vi "Seriennummer zerlegen in Werte.vi"(8 "error in (no error)":errorcluster caption="Fehler (Eingang, kein Fehler)", 10 "Seriennummer":string, 11 "Steuerung PNS Eingang":refnum<class "Steuerung PNS.lvclass">) -> (0 "error out":errorcluster caption="Fehler (Ausgang)", 2 "Werte Array":u16[](array[numeric]), 3 "Steuerung PNS Ausgang":refnum<class "Steuerung PNS.lvclass">)   [LabVIEW 2020, in "Steuerung PNS.lvclass"]
uses:
  Steuerung PNS.lvclass
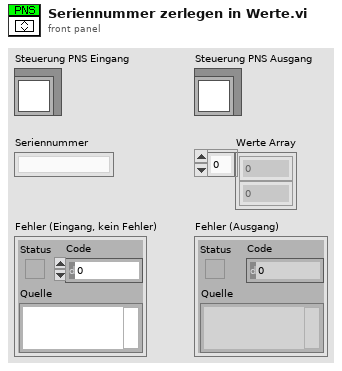
[diagram p1: front panel]
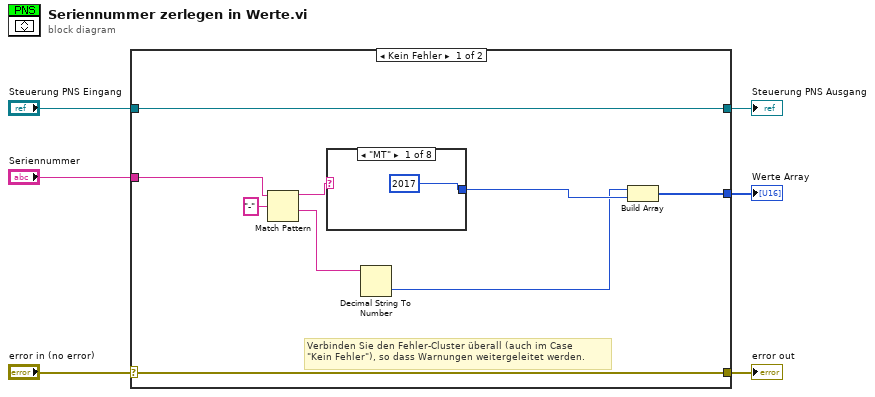
[diagram p0: block diagram]
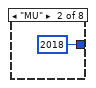
[diagram p2: hidden frame]
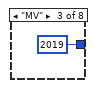
[diagram p3: hidden frame]
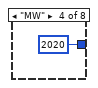
[diagram p4: hidden frame]
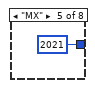
[diagram p5: hidden frame]
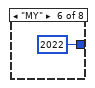
[diagram p6: hidden frame]
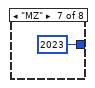
[diagram p7: hidden frame]
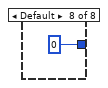
[diagram p8: hidden frame]
diagram:
  n1 = case shown="Kein Fehler" "error in (no error)" {
    selector: "error in (no error)" -> [w14 w25]
    tunnel: [w14 w25] -> w5
    tunnel: [w15 w24] -> w3
    tunnel: "Steuerung PNS Eingang" -> [w15 w24]
    tunnel: "Seriennummer" -> [w12 _]
    tunnel: [w9 _] -> w1
    frame No Error {
      # "Verbinden Sie den Fehler-Cluster überall (auch im Case\n\"Kein Fehler\"), so dass Warnungen weitergeleitet werden."
      n2 = Match Pattern(string=w12, regular expression="-" ("Regulärer Ausdruck")) -> (before substring=w11:string, after substring=w10:string)  [unwired: 1 in, 2 out]
      n3 = case shown="\"MT\"" w11 {
        tunnel: [2017 2018 2019 2020 2021 2022 2023 0] -> w8
        frame "MT" {
        }
        frame "MU" {
        }
        frame "MV" {
        }
        frame "MW" {
        }
        frame "MX" {
        }
        frame "MY" {
        }
        frame "MZ" {
        }
        frame Default {
        }
      }
      n4 = Decimal String To Number(string=w10) -> (number=w7:i32)  [unwired: 2 in, 1 out]
      n5 = Build Array(w7, w8) -> (w9:i32[])
    }
    frame Error {
    }
  }
  "error out" <- w5
  "Steuerung PNS Ausgang" <- w3
  "Werte Array" <- w1
